vi "Move To Position.vi"(6 "Timeout":i32=5000 caption="Timeout (ms)", 8 "error in (no error)":errorcluster, 9 "Velocity (%)":u8=100, 10 "SetPoint":u32, 11 "FHPP in":refnum<class "FHPP.lvclass">) -> (0 "error out":errorcluster, 1 "TimeOut":bool, 2 "Done":bool, 3 "FHPP out":refnum<class "FHPP.lvclass">)   [LabVIEW 2022 SP3, in "FHPP.lvclass"]
uses:
  FHPP.lvclass
  TypeDefs/Operating Mode.ctl
  <vilib>/GPower/Timing/Library/Remaining/Remaining_ms.vi
  <vilib>/GPower/Timing/GPTiming.lvlib
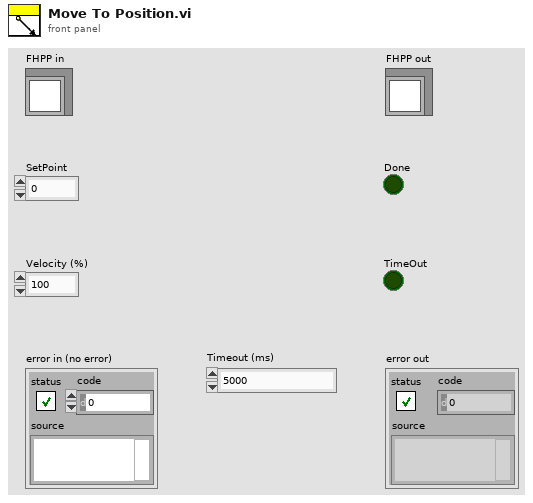
[diagram p1: front panel]
types:
  T1 = typedef "FHPP.lvclass/Operating Mode.ctl" = enum16{"Record Selection", "Direct Mode", "Reserved 1", "Reserved 2"}
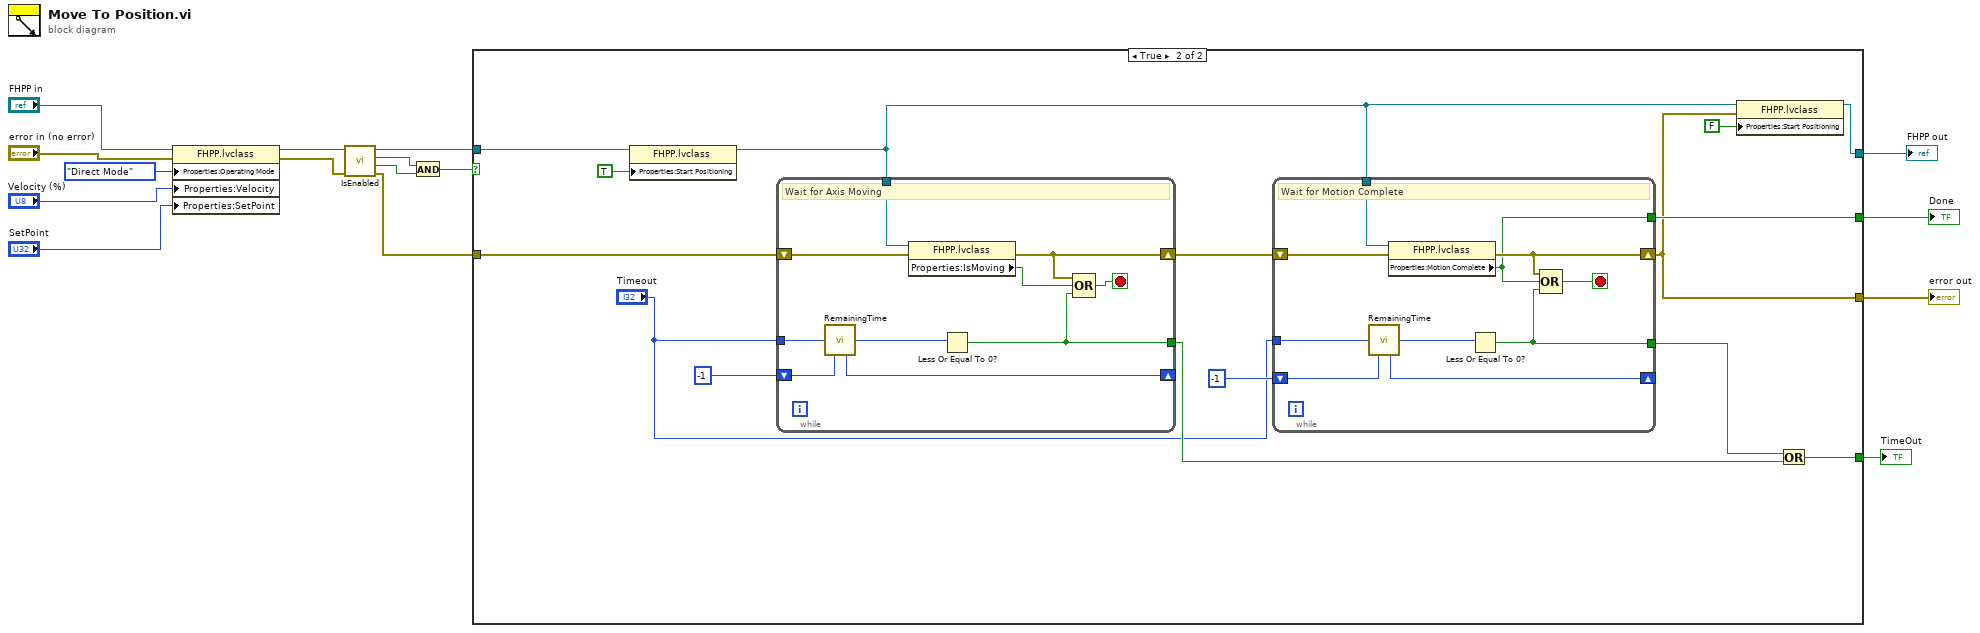
[diagram p0: block diagram]
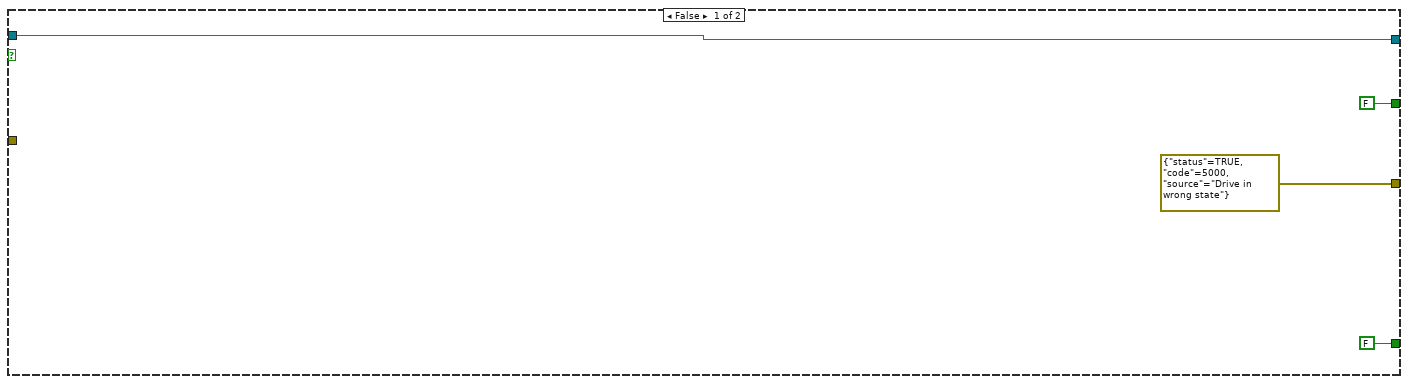
[diagram p2: hidden frame]
diagram:
  n1 = property class="FHPP.lvclass"(reference="FHPP in", error in="error in (no error)", "Properties:Operating Mode"=Operating_Mode."Direct Mode" ("Operating Mode"), "Properties:Velocity"="Velocity (%)", "Properties:SetPoint"="SetPoint") -> (reference out=w2:refnum<class "FHPP.lvclass">, error out=w9:errorcluster)
  n2 = call-dynamic "IsEnabled.vi"("error in (no error)"=w9, "FHPP in"=w2) -> ("error out"=w8:errorcluster, "Operation Enabled"=w5:bool, "Drive Enabled"=w6:bool, "FHPP out"=w1:refnum<class "FHPP.lvclass">)  [unwired: 6 in]
  n3 = And(x=w6, y=w5) -> (x .and. y?=w7:bool)
  n4 = case shown="True" w7 {
    tunnel: w8 -> [_ w35]
    tunnel: [FALSE w29] -> w11
    tunnel: w1 -> [w20 w28]
    tunnel: [w20 w27] -> w10
    tunnel: [FALSE ("Properties:Motion Complete") w22] -> w4
    tunnel: [errorcluster {"status"=TRUE, "code"=5000, "source"="Drive in wrong state"} ("error out") w21] -> w3
    frame False {
    }
    frame True {
      n5 = property class="FHPP.lvclass"(reference=w28, "Properties:Start Positioning"=TRUE ("Start Positioning")) -> (reference out=w25:refnum<class "FHPP.lvclass">)  [unwired: 1 in, 1 out]
      n6 = while {
        tunnel: w25 -> [w55]
        shift-right: [w51] -> w34
        shift-left: w35 -> [w53]
        tunnel: "Timeout" -> [w50]
        shift-right: [w48] -> _
        shift-left: i64 -1 ("Start time in") -> [w49]
        tunnel: [w46] -> w30
        stop <- w52 stop-if-true
        # "Wait for Axis Moving"
        n7 = call-poly <vilib>:"RemainingTime.vi"("Time period target"=w50, "Start time in"=w49) -> ("Remaining time"=w47:i32, "Start time out"=w48:i64)  [unwired: 9 in, 3 out]
        n8 = property class="FHPP.lvclass"(reference=w55, error in=w53) -> (error out=w51:errorcluster, "Properties:IsMoving"=w54:bool)  [unwired: 1 out]
        n9 = Less Or Equal To 0?(x=w47) -> (x <= 0?=w46:bool)
        n10 = Compound Arithmetic op=OR(w51, w54, w46) -> (w52:bool)
      }
      n11 = while {
        tunnel: w25 -> [w45]
        shift-right: [w42] -> w21
        shift-left: w34 -> [w44]
        shift-right: [w40] -> _
        shift-left: i64 -1 ("Start time in") -> [w41]
        tunnel: "Timeout" -> [w39]
        tunnel: [w37] -> w31
        tunnel: [w36] -> w22
        stop <- w43 stop-if-true
        # "Wait for Motion Complete"
        n12 = call-poly <vilib>:"RemainingTime.vi"("Time period target"=w39, "Start time in"=w41) -> ("Remaining time"=w38:i32, "Start time out"=w40:i64)  [unwired: 9 in, 3 out]
        n13 = property class="FHPP.lvclass"(reference=w45, error in=w44) -> (error out=w42:errorcluster, "Properties:Motion Complete"=w36:bool)  [unwired: 1 out]
        n14 = Less Or Equal To 0?(x=w38) -> (x <= 0?=w37:bool)
        n15 = Compound Arithmetic op=OR(w42, w36, w37) -> (w43:bool)
      }
      n16 = property class="FHPP.lvclass"(reference=w25, error in=w21, "Properties:Start Positioning"=FALSE ("Start Positioning")) -> (reference out=w27:refnum<class "FHPP.lvclass">)  [unwired: 1 out]
      n17 = Or(x=w31, y=w30) -> (x .or. y?=w29:bool)
    }
  }
  "FHPP out" <- w10
  "TimeOut" <- w11
  "Done" <- w4
  "error out" <- w3
